vi "Camera.vi"() -> ()   [LabVIEW 2016]
uses:
  Dropbox/Programming/LabVIEW/SPIM Controller/controls/Microscope Settings.ctl
  Dropbox/Programming/LabVIEW/SPIM Controller/controls/CameraControlTypeDef.ctl
  Dropbox/Programming/LabVIEW/SPIM Controller/controls/Stack_State.ctl
  Dropbox/Programming/LabVIEW/SPIM Controller/controls/Stack Track.ctl
  Dropbox/Programming/LabVIEW/SPIM Controller/controls/ModeEnum.ctl
panel:
  in  "Microscope Settings":T1={"Mode"=enum."XY", "Slit"={"Scanning Mode"=12.0, "Slit Width /%"=5.0}, "Colour"=[{"Laser"=enum."561", "Filter"=4}], "Exposure/ms"=40.0, "Piezo Position /um"=0.0, "ROI"={"X"={"Start /px"=0.0, "Step /px"=1.0, "Range /px"=2048.0}, "Y"={"Start /px"=0.0, "Step /px"=1.0, "Range /px"=2048.0}, "Z "={"Start /um"=0.0, "Step/um"=1.0, "Range /um"=100.0}, "T "={"Start /s"=0.0, "Step /s"=1.0, "Range /s"=100.0}}, "Samples per millisecond"=100.0, "Relax/ms"=10.0, "Readout Direction"=2.0, "Trigger Source"=2.0, "Camera Delay /ms"=11.0, "Under Scan /ms"=5.0, "Calibration Coordinates"={"Top Left"=[-4.418670520231216, -0.1592138728323702, 10.0], "Top Right"=[-9.501965317919073, -0.1592138728323702, 10.0], "Bottom Left"=[-4.4508670520231215, 0.0, 0.0], "Bottom Right"=[-9.53757225433526, 0.0, 0.0], "Waveforms"={"Analogue Out"=[], "Digital Out"=[]}}} {"Under Scan /ms" min=0.0 max=10.0 step=0.05; "ROI"."T"."Range /s" min=0.0 max=10.0 step=0.05 format="%<%H:%M:%S>t"; "ROI"."T"."Step /s" min=0.0 max=10.0 step=0.05 format="%<%M:%S%2u>t"; "ROI"."T"."Start /s" min=0.0 max=10.0 step=0.05 format="%<%M:%S%2u>t"; "ROI"."X"."Range /px" min=0.0 max=10.0 step=0.05; "ROI"."X"."Step /px" min=0.0 max=10.0 step=0.05; "ROI"."X"."Start /px" min=0.0 max=10.0 step=0.05; "ROI"."Y"."Range /px" min=0.0 max=10.0 step=0.05; "ROI"."Y"."Step /px" min=0.0 max=10.0 step=0.05; "ROI"."Y"."Start /px" min=0.0 max=10.0 step=0.05; "ROI"."Z"."Range /um" min=0.0 max=10.0 step=0.05; "ROI"."Z"."Step/um" min=0.0001 max=10.0 step=0.05; "ROI"."Z"."Start /um" min=0.0 max=10.0 step=0.05; "Colour"."Filter" items=["Empty"=1, ""=2, ""=3, "561"=4, ""=5, "488"=6]; "Camera Delay /ms" min=0.0 max=10.0 step=0.05; "Trigger Source" items=["Internal"=1.0, "External"=2.0]; "Readout Direction" items=["Forward"=1.0, "Backward"=2.0]; "Slit"."Scanning Mode" items=["Full Frame"=1.0, "Slit Scanning"=12.0]; "Piezo Position /um" min=0.0 max=10.0 step=0.05}
  in  "stop":bool
  in  "Frames":i32
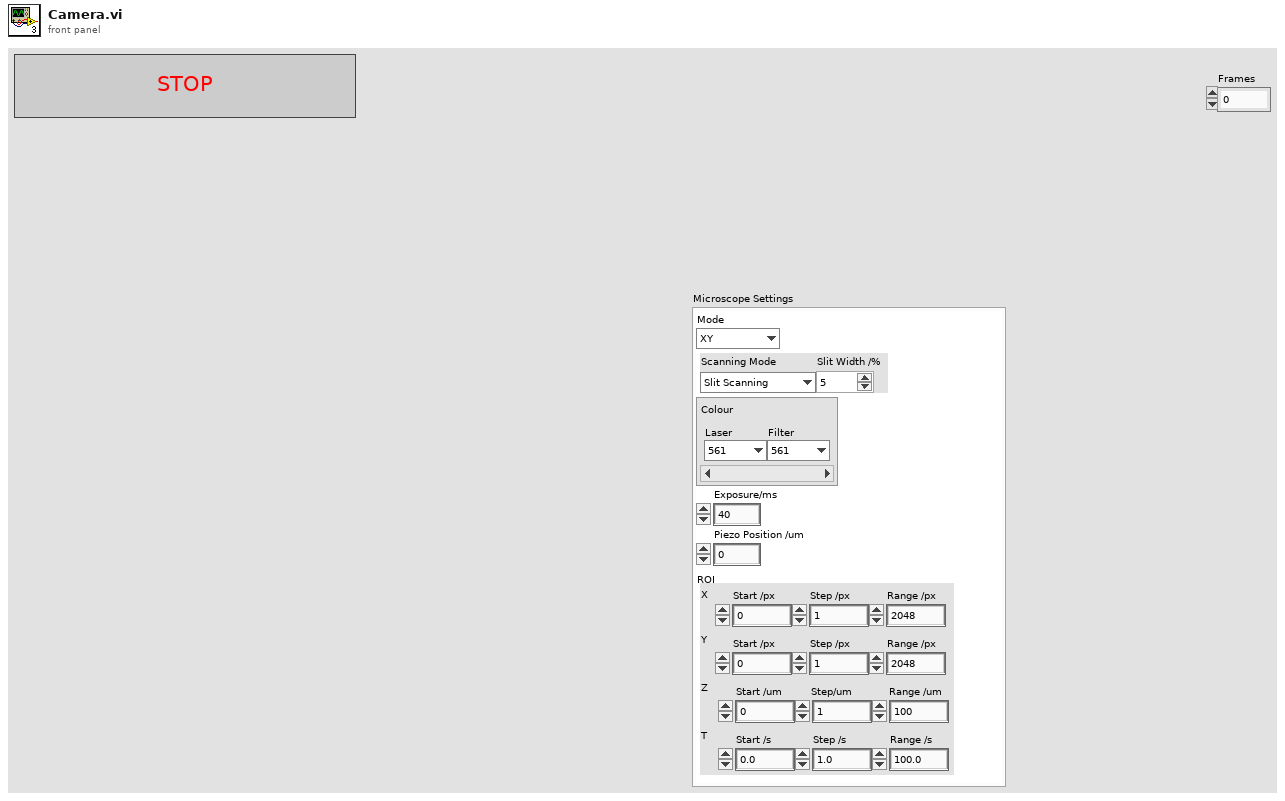
[diagram p1: front panel]
types:
  T1 = typedef "Microscope Settings.ctl" = cluster{"Mode":enum16{"X", "XY", "XYZ", "XYZT", "XYZC", "Tweezers", "Virus"}, "Slit":cluster{"Scanning Mode":dbl, "Slit Width /%":dbl}, "Colour":cluster{"Laser":enum16{"Brightfield", "445", "488", "561", "647"}, "Filter":u16}[], "Exposure/ms":dbl, "Piezo Position /um":dbl, "ROI":cluster{"X":cluster{"Start /px":dbl, "Step /px":dbl, "Range /px":dbl}, "Y":cluster{"Start /px":dbl, "Step /px":dbl, "Range /px":dbl}, "Z ":cluster{"Start /um":dbl, "Step/um":dbl, "Range /um":dbl}, "T ":cluster{"Start /s":dbl, "Step /s":dbl, "Range /s":dbl}}, "Samples per millisecond":dbl, "Relax/ms":dbl, "Readout Direction":dbl, "Trigger Source":dbl, "Camera Delay /ms":dbl, "Under Scan /ms":dbl, "Calibration Coordinates":cluster{"Top Left":dbl[], "Top Right":dbl[], "Bottom Left":dbl[], "Bottom Right":dbl[], "Waveforms":cluster{"Analogue Out":waveform(dbl)[], "Digital Out":digitalwaveform[]}}}
  T2 = cluster{"height":u32, "width":u32, "datatype":u32}
  T3 = typedef "ModeEnum.ctl" = enum16{"Idle", "generateWaves", "runWaves", "runWavesCont", "endWavesCont", "stop"}
  T4 = typedef "Image Type" = u32
  T5 = typedef "Stack_State.ctl" = cluster{"State":T6, "Stack Number":i32, "Image":u16[][], "Stacks":i32}
  T6 = typedef "Stack Track.ctl" = enum16{"Idle", "Display", "Start Sequence", "Read Disk", "STOP", "Collecting", "End", "Save Image"}
  T7 = typedef "CameraControlTypeDef.ctl" = enum16{"Idle", "IntervalLineInt", "Ram Record", "HardDisk Record", "Disengage Update", "Update", "ROI", "Binning", "Scan Mode", "Trigger Mode", "Readout Mode", "Readout Direction", "Preview", "ROIWindow", "Trigger Source"}
  T8 = cluster{"Mode":u32, "Polarity":u32, "Times":u32, "Delay":dbl}
  T9 = cluster{"State":T6, "Timeout":i32, "Data 16":u16[][], "Timeout":i32}
  T10 = enum16{"X", "XY", "XYZ", "XYZT", "XYZC", "Tweezers", "Virus"}
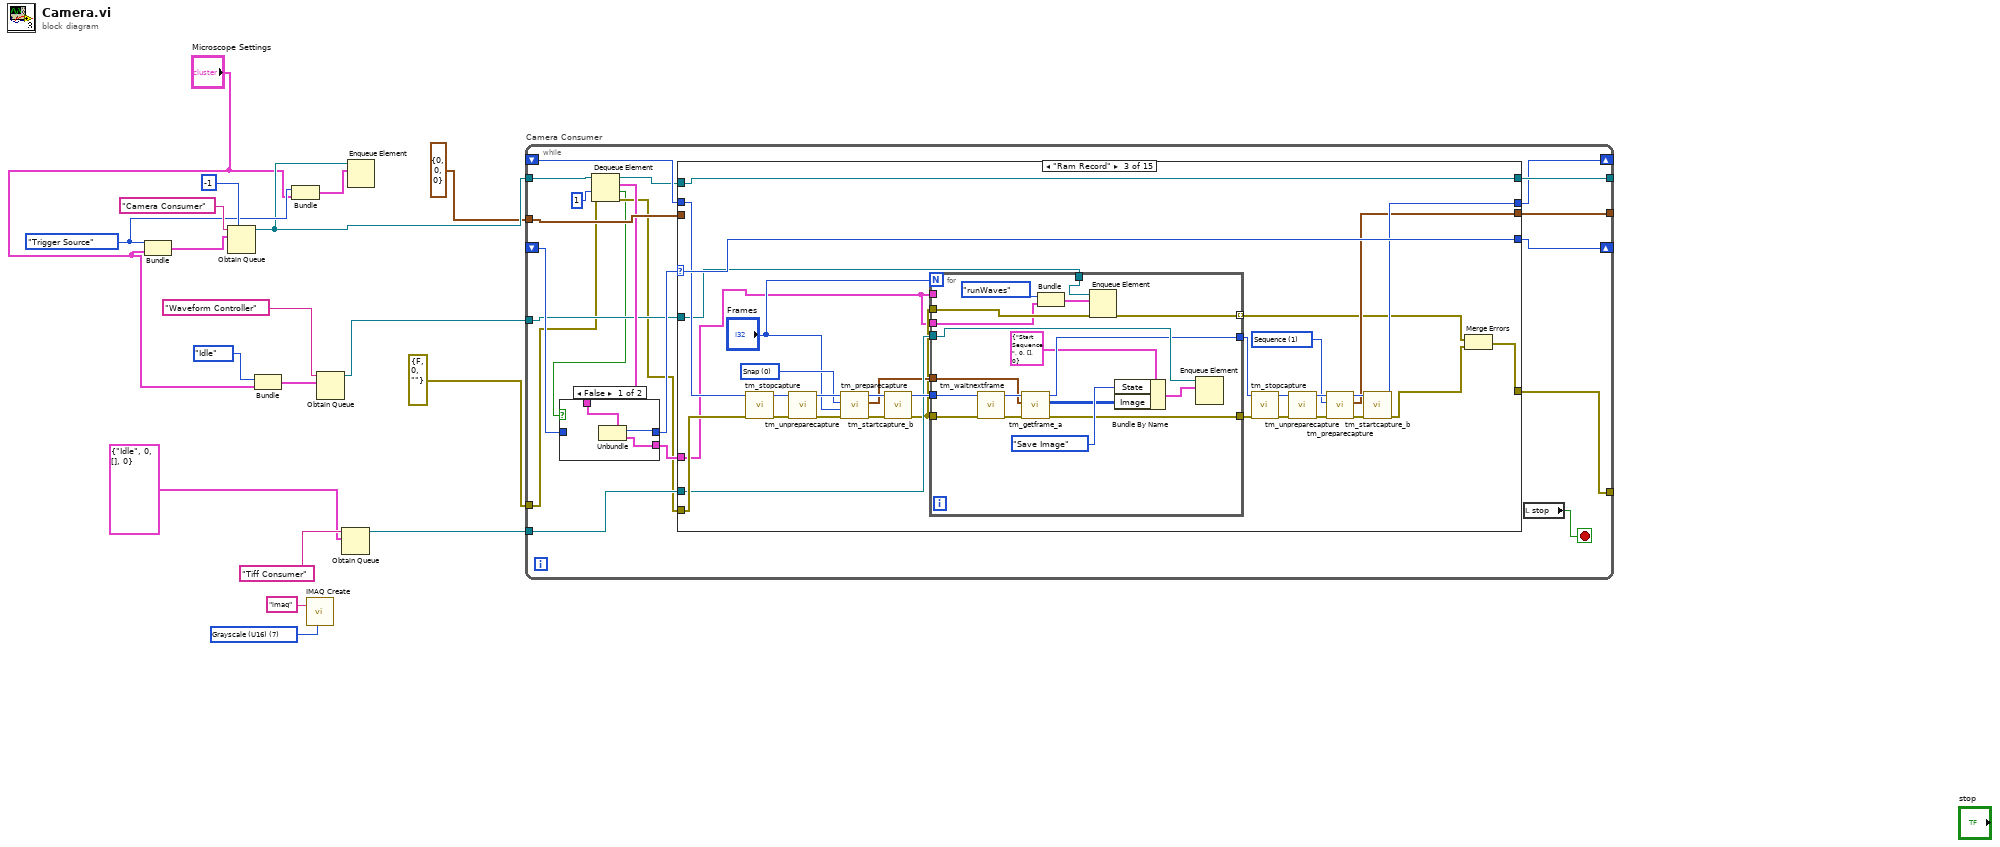
[diagram p0: block diagram]
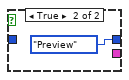
[diagram p2: hidden frame]
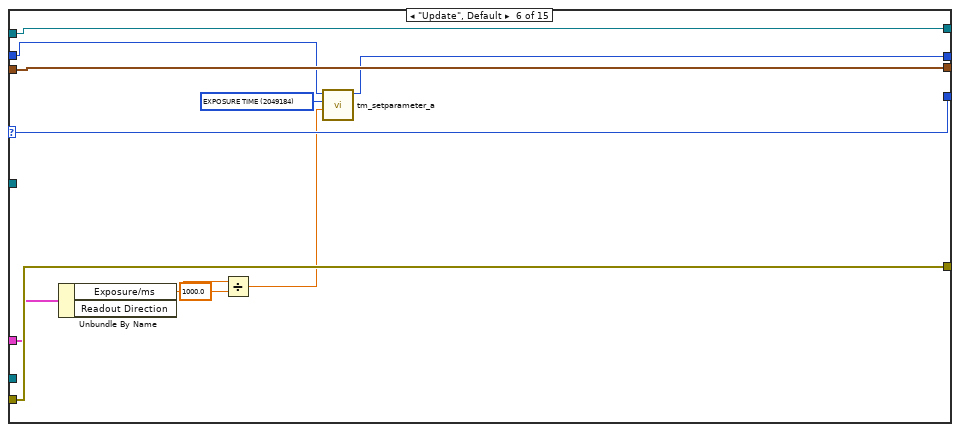
[diagram p7: hidden frame]
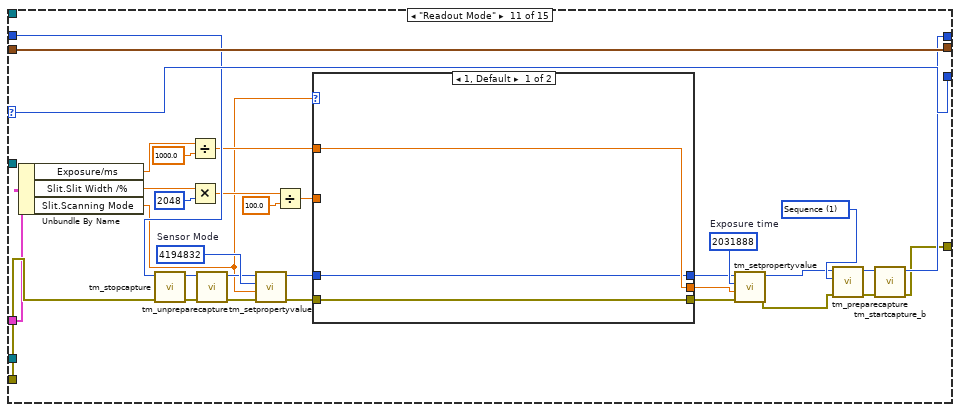
[diagram p12: hidden frame]
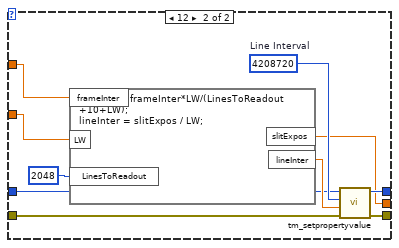
[diagram p13: hidden frame]
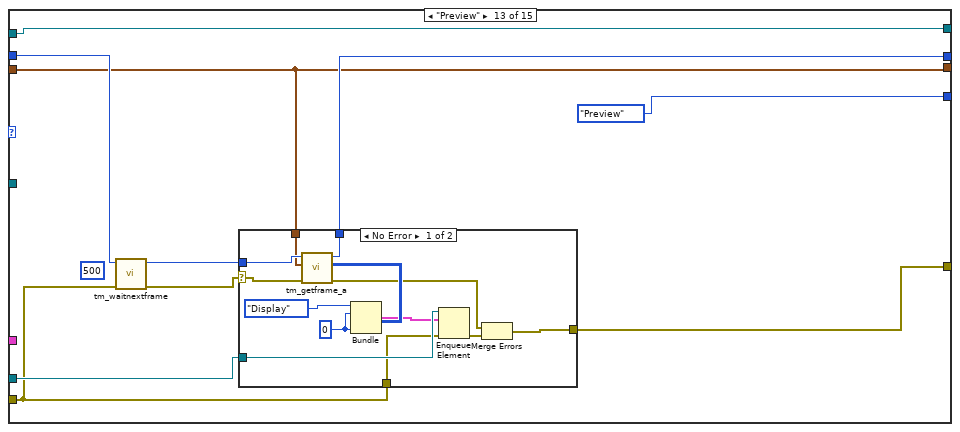
[diagram p15: hidden frame]
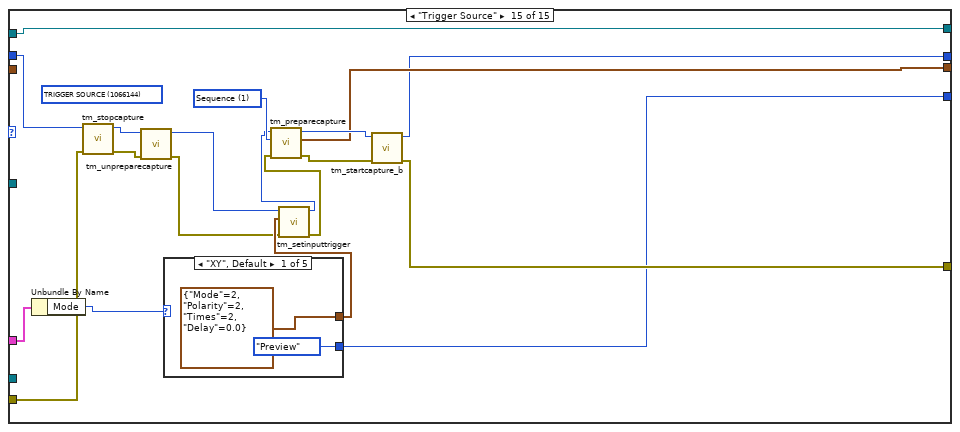
[diagram p18: hidden frame]
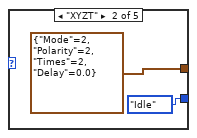
[diagram p19: hidden frame]
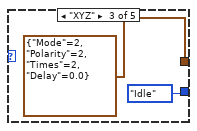
[diagram p20: hidden frame]
diagram:
  w10 = T4 7 items=["Grayscale (U8)", "Grayscale (I16)", "Grayscale (SGL)", "Complex (CSG)", "RGB (U32)", "HSL (U32)", "RGB (U64)", "Grayscale (U16)"] ("Image Type")
  w16 = CameraControlTypeDef."Trigger Source" ("Enum")
  n1 = Bundle("Enum"=w16, "Microscope Settings"="Microscope Settings") -> (w15:cluster{"Enum":T7, "Microscope Settings":T1})  [unwired: 1 in]
  n2 = Obtain Queue(max queue size (-1, unlimited)=-1, name (unnamed)="Camera Consumer", element data type=w15) -> (queue out=w13:refnum<queue>)  [unwired: 2 in, 2 out]
  n3 = Bundle("Mode"=ModeEnum."Idle", "Microscope Settings"="Microscope Settings") -> (w6:cluster{"Mode":T3, "Microscope Settings":T1})  [unwired: 1 in]
  n4 = Bundle("Enum"=w16, "Microscope Settings"="Microscope Settings") -> (w14:cluster{"Enum":T7, "Microscope Settings":T1})  [unwired: 1 in]
  n5 = call "IMAQ Create"("Image Name"="imaq", "Image Type"=w10) -> ()  [unwired: 3 in, 2 out]
  n6 = Obtain Queue(name (unnamed)="Waveform Controller", element data type=w6) -> (queue out=w4:refnum<queue>)  [unwired: 3 in, 2 out]
  n7 = Obtain Queue(name (unnamed)="Tiff Consumer", element data type=T5 {"State"=enum."Idle", "Stack Number"=0, "Image"=[], "Stacks"=0} ("input cluster")) -> (queue out=w8:refnum<queue>)  [unwired: 3 in, 2 out]
  n8 = Enqueue Element(queue=w13, element=w14) -> ()  [unwired: 2 in, 3 out]
  n9 = while "Camera Consumer" {
    tunnel: errorcluster {"status"=FALSE, "code"=0, "source"=""} ("error IO") -> [w20]
    tunnel: [w24] -> _
    tunnel: w13 -> [w31]
    tunnel: [w38] -> _
    shift-right: [w37] -> _
    shift-left: _ -> [w28]
    tunnel: [w34] -> _
    tunnel: T2 {"height"=0, "width"=0, "datatype"=0} ("Buffer Info") -> [w33]
    tunnel: w8 -> [w27]
    shift-right: [w35] -> _
    shift-left: _ -> [w36]
    tunnel: w4 -> [w22]
    stop <- w23 stop-if-true
    n10 = Dequeue Element(queue=w31, timeout in ms (-1)=1, error in (no error)=w20) -> (queue out=w30:refnum<queue>, element=w26:cluster{"Enum":T7, "Microscope Settings":T1}, timed out?=w19:bool, error out=w21:errorcluster)
    n11 = case shown="False" w19 {
      tunnel: [w40 CameraControlTypeDef."Preview" ("Enum")] -> w29
      tunnel: w28 -> [_ _]
      tunnel: w26 -> [w41 _]
      tunnel: [w39 _] -> w25
      frame False {
        n12 = Unbundle(w41) -> ("Enum"=w40:T7, "Microscope Settings"=w39:T1)
      }
      frame True {
      }
    }
    n13 = case shown="\"Ram Record\"" w29 {
      selector: w29 -> [w46 w51 w83 w106 w111 w122 w127 w132 w137 w142 w175 w193 _ w221 _]
      tunnel: w30 -> [w45 w52 w84 w107 w112 w123 w128 w133 w138 w143 _ w189 w203 w223 w242]
      tunnel: [w45 w52 w84 w107 w112 w123 w128 w133 w138 w143 _ w189 w203 w223 w242] -> w38
      tunnel: w21 -> [w47 w50 w82 w105 w110 w121 w126 w131 w136 w141 w170 w192 w196 w220 w233]
      tunnel: [w47 w50 w59 w105 w110 w121 w126 w131 w136 w141 w144 w192 w195 w220 w234] -> w24
      tunnel: [w46 w51 w83 w106 w111 w122 w127 w132 w137 w142 w175 w193 CameraControlTypeDef."Preview" ("Enum") w221 w224] -> w37
      tunnel: w36 -> [w44 w49 w66 w104 w108 w119 w125 w130 w135 w140 w172 w191 w202 w222 w236]
      tunnel: [w44 w49 w65 w104 w108 w118 w125 w130 w135 w140 w146 w191 w200 w222 w235] -> w35
      tunnel: [w43 w48 w61 w103 w109 w120 w124 w129 w134 w139 w174 w190 w198 w219 w237] -> w34
      tunnel: w33 -> [w43 w48 _ w103 w109 w120 w124 w129 w134 w139 w174 w190 w198 w219 _]
      tunnel: w27 -> [_ _ w75 _ _ _ _ _ _ _ _ _ w197 _ _]
      tunnel: w25 -> [_ _ w54 _ _ w117 _ _ _ _ w169 _ _ _ w226]
      tunnel: w22 -> [_ _ w55 _ _ _ _ _ _ _ _ _ _ _ _]
      frame "Idle" {
      }
      frame "IntervalLineInt" {
      }
      frame "Ram Record" {
        w79 = 0 items=["Snap", "Sequence"] ("Capture mode")
        w62 = 1 items=["Snap", "Sequence"] ("Capture mode")
        n14 = call <userlib>:"tm_stopcapture.vi"("error in (no error)"=w82, "Handle in"=w66) -> ("error out"=w57:errorcluster, "Handle out"=w58:u32)  [unwired: 8 in]
        n15 = call <userlib>:"tm_unpreparecapture.vi"("error in (no error)"=w57, "Handle in"=w58) -> ("error out"=w81:errorcluster, "Handle out"=w80:u32)  [unwired: 8 in]
        n16 = call <userlib>:"tm_preparecapture.vi"("error in (no error)"=w81, "Frames"="Frames", "Capture mode"=w79, "Handle in"=w80) -> ("error out"=w77:errorcluster, "Buffer Info"=w63:T2, "Handle out"=w78:u32)  [unwired: 4 in, 1 out]
        n17 = call <userlib>:"tm_startcapture_b.vi"("error in (no error)"=w77, "Handle in"=w78) -> ("error out"=w56:errorcluster, "Handle out"=w76:u32)  [unwired: 8 in]
        n18 = for {
          N: "Frames" -> [_]
          tunnel: w56 -> [w102]
          tunnel: w76 -> [w101]
          tunnel: w75 -> [w97]
          tunnel: [w95] -> w71
          tunnel: [w94] -> w70
          tunnel: w63 -> [w93]
          tunnel: w56 -> [w90]
          tunnel: w55 -> [w89]
          tunnel: w54 -> [_]
          tunnel: w54 -> [w87]
          tunnel: [w86] -> w53 mode=indexing
          n19 = call <userlib>:"tm_waitnextframe.vi"("error in (no error)"=w102, "Handle in"=w101) -> ("error out"=w100:errorcluster, "Handle out"=w99:u32)  [unwired: 6 in, 2 out]
          n20 = call <userlib>:"tm_getframe_a.vi"("error in (no error)"=w100, "Buffer Info"=w93, "Handle in"=w99) -> ("error out"=w95:errorcluster, "Data 16"=w91:u16[][], "Handle out"=w94:u32)  [unwired: 4 in, 2 out]
          n21 = Bundle("Mode"=ModeEnum."runWaves", "Microscope Settings"=w87) -> (w85:cluster{"Mode":T3, "Microscope Settings":T1})  [unwired: 1 in]
          n22 = Enqueue Element(queue=w89, element=w85, error in (no error)=w90) -> (error out=w86:errorcluster)  [unwired: 1 in, 2 out]
          n23 = Bundle By Name(cluster=T5 {"State"=enum."Start Sequence", "Stack Number"=0, "Image"=[], "Stacks"=0} ("element"), "State"=Stack_Track."Save Image", "Image"=w91) -> (w96:T5)
          n24 = Enqueue Element(queue=w97, element=w96) -> ()  [unwired: 2 in, 3 out]
        }
        n25 = call <userlib>:"tm_stopcapture.vi"("error in (no error)"=w71, "Handle in"=w70) -> ("error out"=w72:errorcluster, "Handle out"=w69:u32)  [unwired: 8 in]
        n26 = call <userlib>:"tm_unpreparecapture.vi"("error in (no error)"=w72, "Handle in"=w69) -> ("error out"=w73:errorcluster, "Handle out"=w68:u32)  [unwired: 8 in]
        n27 = call <userlib>:"tm_preparecapture.vi"("error in (no error)"=w73, "Capture mode"=w62, "Handle in"=w68) -> ("error out"=w74:errorcluster, "Buffer Info"=w61:T2, "Handle out"=w67:u32)  [unwired: 5 in, 1 out]
        n28 = call <userlib>:"tm_startcapture_b.vi"("error in (no error)"=w74, "Handle in"=w67) -> ("error out"=w60:errorcluster, "Handle out"=w65:u32)  [unwired: 8 in]
        n29 = Merge Errors(w53, w60) -> (w59:errorcluster)
      }
      frame "HardDisk Record" {
      }
      frame "Disengage Update" {
      }
      frame "Update", Default {
        w114 = u32 2049184 items=["SENSOR MODE"=4212128, "CCD MODE"=4212384, "READOUT MODE"=4211872, "ACTIVE VIEW INDEX"=4343136, "BITS PER CHANNEL"=4342976, "IMAGE PIXEL TYPE"=4343296, "BINNING"=4215968, "EXPOSURE TIME"=2049184, "CONTRAST GAIN"=3163312, "CONTRAST OFFSET"=3163328, "LIGHT MODE"=2114720, "SENSITIVITY"=2114992, "PHOTON IMAGING MODE"=2115200, "HIGH DYNAMIC RANGE MODE"=3163360, "WHITE BALANCE"=3163568, "TEMPERATURE"=2115232, "TEMPERATURE TARGET"=2115264, "SENSOR COOLER FAN"=2115296, "LINEBUNDLE HEIGHT"=4212192, "MECHANICAL SHUTTER"=2115488, "BACK FOCUS POSITION"=8422304, "TRIGGER CONNECTOR"=1066432, "TRIGGER SOURCE"=1066144, "OUTPUT TRIGGER SOURCE"=1852576, "TRIGGER GLOBAL EXPOSURE"=2049680, "FIRST TRIGGER BEHAVIOR"=2049696, "CHANNEL SYNC"=1852352, "READOUT DIRECTION"=4211904, "PRE HSYNC COUNT"=1852704, "INTERNAL LINE SPEED"=4226000, "INTERNAL LINE INTERVAL"=4226016] ("Parameter")
        n30 = Unbundle By Name(w117) -> ("Exposure/ms"=w116:dbl)  [unwired: 1 out]
        n31 = Divide(x=w116, y=1000.0) -> (x/y=w113:dbl)
        n32 = call <userlib>:"tm_setparameter_a.vi"("Value in"=w113, "Parameter"=w114, "Handle in"=w119) -> ("Handle out"=w118:u32)  [unwired: 7 in, 1 out]
      }
      frame "ROI" {
      }
      frame "Binning" {
      }
      frame "Scan Mode" {
      }
      frame "Trigger Mode" {
      }
      frame "Readout Mode" {
        w150 = 1 items=["Snap", "Sequence"] ("Capture mode")
        w156 = u32 4194832  # Sensor Mode
        w159 = u32 2031888  # Exposure time
        n33 = Unbundle By Name(w169) -> ("Exposure/ms"=w168:dbl, "Slit.Slit Width /%"=w164:dbl, "Slit.Scanning Mode"=w154:dbl)
        n34 = call <userlib>:"tm_stopcapture.vi"("error in (no error)"=w170, "Handle in"=w172) -> ("error out"=w173:errorcluster, "Handle out"=w171:u32)  [unwired: 8 in]
        n35 = Divide(x=w168, y=1000.0) -> (x/y=w166:dbl)
        n36 = Multiply(x=w164, y=2048 ("input variable")) -> (x*y=w163:dbl)
        n37 = call <userlib>:"tm_unpreparecapture.vi"("error in (no error)"=w173, "Handle in"=w171) -> ("error out"=w151:errorcluster, "Handle out"=w155:u32)  [unwired: 8 in]
        n38 = call "tm_setpropertyvalue.vi"("error in (no error)"=w151, "Value in"=w154, "Property ID"=w156, "Handle in"=w155) -> ("error out"=w152:errorcluster, "Handle out"=w153:u32)  [unwired: 6 in]
        n39 = Divide(x=w163, y=100.0) -> (x/y=w161:dbl)
        n40 = case shown="1, Default" w154 {
          tunnel: [w178 w179] -> w160
          tunnel: w166 -> [w178 w187]
          tunnel: w161 -> [_ w186]
          tunnel: w153 -> [w177 w181]
          tunnel: [w177 w183] -> w158
          tunnel: [w176 w182] -> w157
          tunnel: w152 -> [w176 w180]
          frame 1, Default {
          }
          frame 12 {
            w185 = u32 4208720  # Line Interval
            n41 = formula code="slitExpos=frameInter*LW/(LinesToReadout\n+10+LW);\nlineInter = slitExpos / LW;"("frameInter"=w187, "LW"=w186, "LinesToReadout"=2048 ("input variable")) -> ("slitExpos"=w179:dbl, "lineInter"=w184:dbl)
            n42 = call "tm_setpropertyvalue.vi"("error in (no error)"=w180, "Value in"=w184, "Property ID"=w185, "Handle in"=w181) -> ("error out"=w182:errorcluster, "Handle out"=w183:u32)  [unwired: 6 in]
          }
        }
        n43 = call "tm_setpropertyvalue.vi"("error in (no error)"=w157, "Value in"=w160, "Property ID"=w159, "Handle in"=w158) -> ("error out"=w145:errorcluster, "Handle out"=w147:u32)  [unwired: 6 in]
        n44 = call <userlib>:"tm_preparecapture.vi"("error in (no error)"=w145, "Capture mode"=w150, "Handle in"=w147) -> ("error out"=w149:errorcluster, "Handle out"=w148:u32)  [unwired: 5 in, 2 out]
        n45 = call <userlib>:"tm_startcapture_b.vi"("error in (no error)"=w149, "Handle in"=w148) -> ("error out"=w144:errorcluster, "Handle out"=w146:u32)  [unwired: 8 in]
      }
      frame "Readout Direction" {
      }
      frame "Preview" {
        (unwired) 500 ("Timeout")
        n46 = call <userlib>:"tm_waitnextframe.vi"("error in (no error)"=w196, "Handle in"=w202) -> ("error out"=w194:errorcluster, "Handle out"=w201:u32)  [unwired: 6 in, 2 out]
        n47 = case shown="No Error" w194 {
          selector: w194 -> [w204 w218]
          tunnel: w201 -> [w216 w217]
          tunnel: [w215 w217] -> w200
          tunnel: w198 -> [w214 _]
          tunnel: w197 -> [w213 _]
          tunnel: w196 -> [w208 _]
          tunnel: [w205 w218] -> w195
          frame No Error {
            w210 = 0 ("Timeout")
            n48 = call <userlib>:"tm_getframe_a.vi"("error in (no error)"=w204, "Buffer Info"=w214, "Handle in"=w216) -> ("error out"=w206:errorcluster, "Data 16"=w211:u16[][], "Handle out"=w215:u32)  [unwired: 4 in, 2 out]
            n49 = Bundle("State"=Stack_Track."Display", "Timeout"=w210, "Data 16"=w211, "Timeout"=w210) -> (w209:T9)  [unwired: 1 in]
            n50 = Enqueue Element(queue=w213, element=w209, error in (no error)=w208) -> (error out=w207:errorcluster)  [unwired: 1 in, 2 out]
            n51 = Merge Errors(w206, w207) -> (w205:errorcluster)
          }
          frame Error {
          }
        }
      }
      frame "ROIWindow" {
      }
      frame "Trigger Source" {
        (unwired) u32 1066144 items=["SENSOR MODE"=4212128, "CCD MODE"=4212384, "READOUT MODE"=4211872, "ACTIVE VIEW INDEX"=4343136, "BITS PER CHANNEL"=4342976, "IMAGE PIXEL TYPE"=4343296, "BINNING"=4215968, "EXPOSURE TIME"=2049184, "CONTRAST GAIN"=3163312, "CONTRAST OFFSET"=3163328, "LIGHT MODE"=2114720, "SENSITIVITY"=2114992, "PHOTON IMAGING MODE"=2115200, "HIGH DYNAMIC RANGE MODE"=3163360, "WHITE BALANCE"=3163568, "TEMPERATURE"=2115232, "TEMPERATURE TARGET"=2115264, "SENSOR COOLER FAN"=2115296, "LINEBUNDLE HEIGHT"=4212192, "MECHANICAL SHUTTER"=2115488, "BACK FOCUS POSITION"=8422304, "TRIGGER CONNECTOR"=1066432, "TRIGGER SOURCE"=1066144, "OUTPUT TRIGGER SOURCE"=1852576, "TRIGGER GLOBAL EXPOSURE"=2049680, "FIRST TRIGGER BEHAVIOR"=2049696, "CHANNEL SYNC"=1852352, "READOUT DIRECTION"=4211904, "PRE HSYNC COUNT"=1852704, "INTERNAL LINE SPEED"=4226000, "INTERNAL LINE INTERVAL"=4226016] ("Parameter")
        w232 = 1 items=["Snap", "Sequence"] ("Capture mode")
        n52 = Unbundle By Name(w226) -> ("Mode"=w225:T10)
        n53 = call <userlib>:"tm_stopcapture.vi"("error in (no error)"=w233, "Handle in"=w236) -> ("error out"=w240:errorcluster, "Handle out"=w241:u32)  [unwired: 8 in]
        n54 = call <userlib>:"tm_unpreparecapture.vi"("error in (no error)"=w240, "Handle in"=w241) -> ("error out"=w228:errorcluster, "Handle out"=w231:u32)  [unwired: 8 in]
        n55 = case shown="\"XY\", Default" w225 {
          tunnel: [T8 {"Mode"=2, "Polarity"=2, "Times"=2, "Delay"=0.0} ("Parameters") T8 {"Mode"=2, "Polarity"=2, "Times"=2, "Delay"=0.0} ("Parameters") T8 {"Mode"=2, "Polarity"=2, "Times"=2, "Delay"=0.0} ("Parameters") T8 {"Mode"=1, "Polarity"=2, "Times"=2, "Delay"=0.0} ("Parameters") T8 {"Mode"=1, "Polarity"=2, "Times"=2, "Delay"=0.0} ("Parameters")] -> w229
          tunnel: [CameraControlTypeDef."Preview" ("Enum") CameraControlTypeDef."Idle" ("Enum") CameraControlTypeDef."Idle" ("Enum") CameraControlTypeDef."Idle" ("Enum") CameraControlTypeDef."Preview" ("Enum")] -> w224
          frame "XY", Default {
          }
          frame "XYZT" {
          }
          frame "XYZ" {
          }
          frame "XYZC" {
          }
          frame "X" {
          }
        }
        n56 = call <userlib>:"tm_setinputtrigger.vi"("error in (no error)"=w228, "Parameters"=w229, "Handle in"=w231) -> ("error out"=w227:errorcluster, "Handle out"=w230:u32)  [unwired: 7 in]
        n57 = call <userlib>:"tm_preparecapture.vi"("error in (no error)"=w227, "Capture mode"=w232, "Handle in"=w230) -> ("error out"=w239:errorcluster, "Buffer Info"=w237:T2, "Handle out"=w238:u32)  [unwired: 5 in, 1 out]
        n58 = call <userlib>:"tm_startcapture_b.vi"("error in (no error)"=w239, "Handle in"=w238) -> ("error out"=w234:errorcluster, "Handle out"=w235:u32)  [unwired: 8 in]
      }
    }
    n59 = local read "stop"() -> (w23:bool)
  }
